vi "email.vi"(9 "Plant Method":T1={"Operator information"=[], "data log interval"=60, "data loop interval"=10, "Datalog directory path"=path "", "graph update interval"=1.0, "history length"=1000, "Control Logic file path"=path "", "Sensor Configuration file path"=path "", "HMI VI path"=path "", "HMI data smooth"=5.0} {"HMI data smooth" min=0.01 format="%.2f"; "history length" min=1; "graph update interval" min=0.1 format="%.2f"; "data log interval" min=1}, 10 "message":string, 11 "subject":string) -> ()   [LabVIEW 2012]
uses:
  Plant method.ctl
  operator info.ctl
  <vilib>/Utility/SMTP/NI_SMTPEmail.lvlib
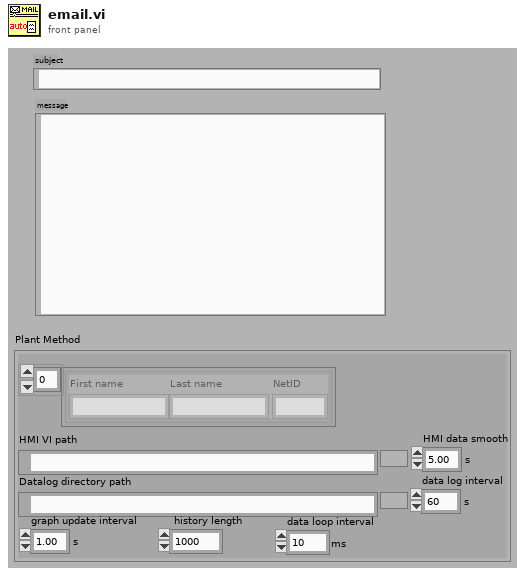
[diagram p1: front panel]
types:
  T1 = typedef "Plant method.ctl" = cluster{"Operator information":T2, "data log interval":u32, "data loop interval":u32, "Datalog directory path":path, "graph update interval":sgl, "history length":u16, "Control Logic file path":path, "Sensor Configuration file path":path, "HMI VI path":path, "HMI data smooth":dbl}
  T2 = typedef "operator info.ctl" = cluster{"First name":string, "Last name":string, "NetID":string}[]
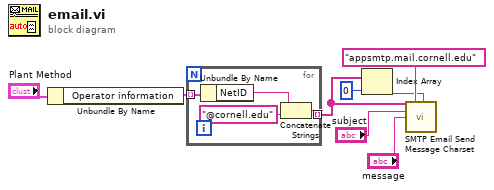
[diagram p0: block diagram]
diagram:
  n1 = Unbundle By Name("Plant Method") -> ("Operator information"=w7:T2)
  n2 = for {
    tunnel: w7 -> [w9] mode=indexing
    tunnel: [w10] -> w6 mode=indexing
    n3 = Unbundle By Name(w9) -> ("NetID"=w12:string)
    n4 = Concatenate Strings(w12, "@cornell.edu" ("string")) -> (w10:string)
  }
  n5 = Index Array(array=w6, index=0) -> (element=w4:string)
  n6 = call <vilib>:"SMTP Email Send Message Charset.vi"("recipients"=w6, "mail server"="appsmtp.mail.cornell.edu", "return address"=w4, "subject ([No Subject])"="subject", "message"="message") -> ()  [unwired: 9 in, 2 out]
